vi "generatore_dente_sega_-1_1.vi"(0 "f0 (frequenza base) [Hz]":dbl min=0.0, 1 "Ap (ampiezza di picco)":dbl min=0.0, 2 "Tc (periodo di campionamento) [s]":dbl min=0.0, 3 "Ta (tempo di analisi) [s]":dbl min=0.0, 5 "Phi (fase iniziale) [rad]":dbl, 8 "DC Offset":dbl) -> (7 "Waveform Graph":waveform(dbl)(graph))   [LabVIEW 2009]
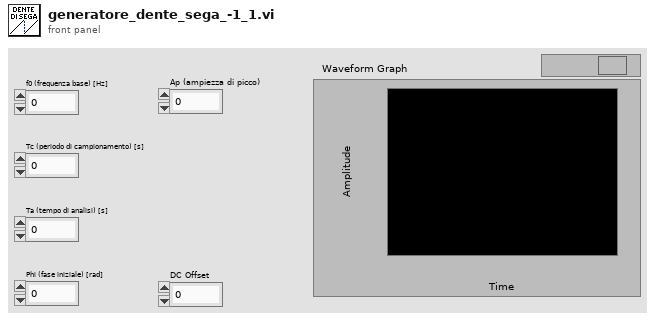
[diagram p1: front panel]
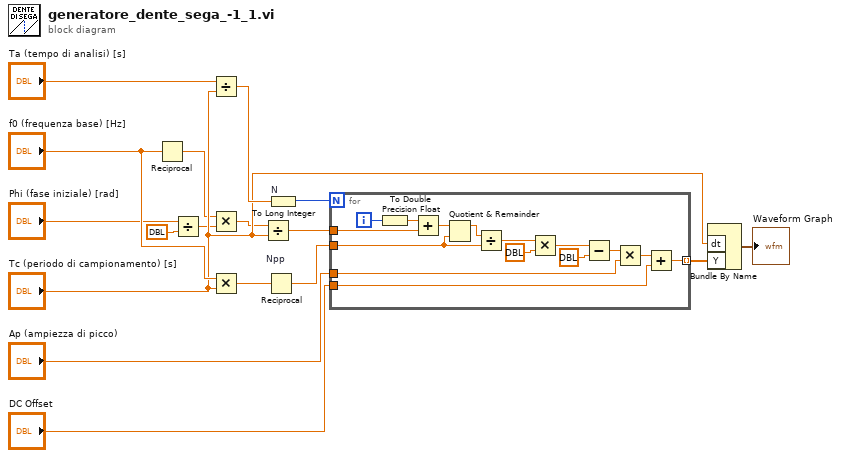
[diagram p0: block diagram]
diagram:
  n1 = Reciprocal(x="f0 (frequenza base) [Hz]") -> (1/x=w6:dbl)
  n2 = Divide(x="Phi (fase iniziale) [rad]", y=dbl ?) -> (x/y=w5:dbl)
  n3 = Divide(x="Ta (tempo di analisi) [s]", y="Tc (periodo di campionamento) [s]") -> (x/y=w11:dbl)
  n4 = Multiply(x=w6, y=w5) -> (x*y=w2:dbl)
  n5 = Multiply(x="f0 (frequenza base) [Hz]", y="Tc (periodo di campionamento) [s]") -> (x*y=w16:dbl)
  n6 = Divide(x=w2, y="Tc (periodo di campionamento) [s]") -> (x/y=w1:dbl)
  n7 = Reciprocal "Npp"(x=w16) -> (1/x=w17:dbl)
  n8 = To Long Integer "N"(number=w11) -> (32bit integer=w12:i32)
  n9 = for {
    N: w12 -> [_]
    tunnel: "DC Offset" -> [w29]
    tunnel: "Ap (ampiezza di picco)" -> [w31]
    tunnel: [w28] -> w9 mode=indexing
    tunnel: w17 -> [w27]
    tunnel: w1 -> [w18]
    i -> [w26]
    n10 = To Double Precision Float(number=w26) -> (double precision float=w24:dbl)
    n11 = Add(x=w24, y=w18) -> (x+y=w23:dbl)
    n12 = Quotient & Remainder(x=w23, y=w27) -> (x-y*floor(x/y)=w25:dbl)  [unwired: 1 out]
    n13 = Divide(x=w25, y=w27) -> (x/y=w22:dbl)
    n14 = Multiply(x=w22, y=dbl ?) -> (x*y=w20:dbl)
    n15 = Subtract(x=w20, y=dbl ?) -> (x-y=w32:dbl)
    n16 = Multiply(x=w32, y=w31) -> (x*y=w30:dbl)
    n17 = Add(x=w30, y=w29) -> (x+y=w28:dbl)
  }
  n18 = Bundle By Name("dt"="Tc (periodo di campionamento) [s]", "Y"=w9) -> (→"Waveform Graph":waveform(dbl))  [unwired: 1 in]
